vi "Chi-Squared Random.vi"(6 "seed":i32=-1, 7 "reset":bool, 10 "k":i32=1, 11 "samples":i32=128) -> (0 "error":i32, 3 "chi-squared random data":dbl[](array[numeric]))   [LabVIEW 2017, in "NI_Gmath.lvlib"]
doc: "Generates random values from a variate X, where X describes the selected distribution type. You must manually select the polymorphic instance to use."
uses:
  <vilib>/gmath/NI_Gmath.lvlib
panel:
  # "Chi-Squared Random"
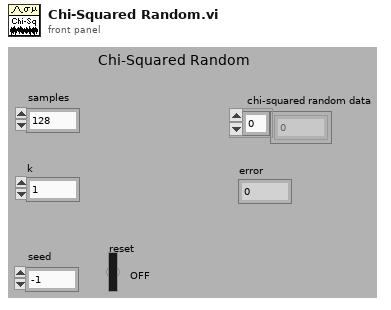
[diagram p1: front panel]
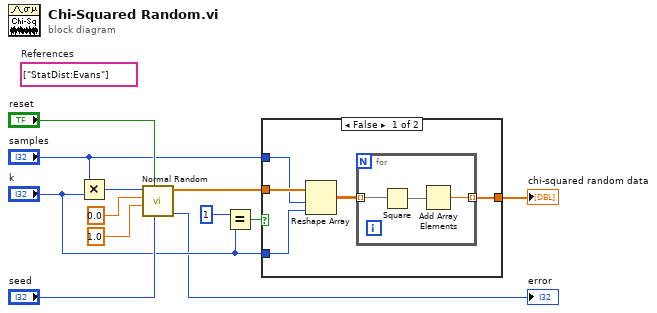
[diagram p0: block diagram]
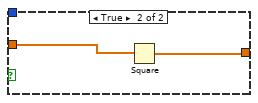
[diagram p2: hidden frame]
diagram:
  (unwired) string[] ["StatDist:Evans"]  # References
  n1 = Multiply(x="samples", y="k") -> (x*y=w8:i32)
  n2 = call <vilib>:"Normal Random.vi"("seed"="seed", "reset"="reset", "std"=1.0, "mean"=0.0, "samples"=w8) -> ("error"=→"error":i32, "normal random data"=w7:dbl[])  [unwired: 5 in]
  n3 = Equal?(x=1 ("y"), y="k") -> (x = y?=w2:bool)
  n4 = case shown="False" w2 {
    tunnel: w7 -> [w17 w22]
    tunnel: "samples" -> [w16 _]
    tunnel: "k" -> [w15 _]
    tunnel: [w13 w21] -> w5
    frame False {
      n5 = Reshape Array(w17, w16, w15) -> (w14:dbl[][])
      n6 = for {
        tunnel: w14 -> [w20] mode=indexing
        tunnel: [w18] -> w13 mode=indexing
        n7 = Square(x=w20) -> (x^2=w19:dbl[])
        n8 = Add Array Elements(numeric array=w19) -> (sum=w18:dbl)
      }
    }
    frame True {
      n9 = Square(x=w22) -> (x^2=w21:dbl[])
    }
  }
  "chi-squared random data" <- w5
